vi "checkAllBridgesTested.vi"(8 "error in (no error)":errorcluster, 11 "TestMonitor in":refnum<class "TestMonitor.lvclass">) -> (0 "error out":errorcluster, 2 "allBridgesTestedIsTrue":bool, 3 "TestMonitor out":refnum<class "TestMonitor.lvclass">)   [LabVIEW 2013, in "TestMonitor.lvclass"]
uses:
  TestMonitor.lvclass
  TestMonitor.lvclass/TestMonitor.ctl
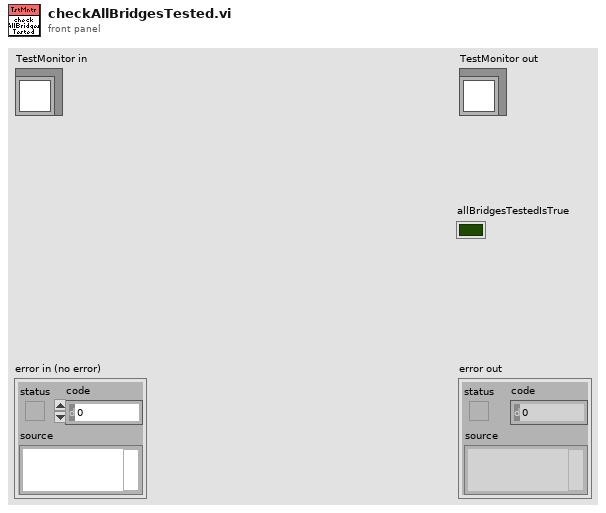
[diagram p1: front panel]
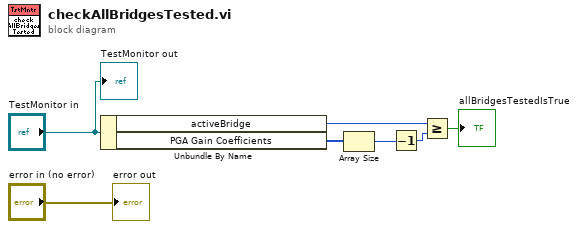
[diagram p0: block diagram]
diagram:
  n1 = Unbundle By Name("TestMonitor in") -> ("activeBridge"=w3:u32, "PGA Gain Coefficients"=w5:u8[])
  n2 = Array Size(array=w5) -> (size(s)=w4:i32)
  n3 = Decrement(x=w4) -> (x-1=w2:i32)
  n4 = Greater Or Equal?(x=w3, y=w2) -> (x >= y?=→"allBridgesTestedIsTrue":bool)
  "error out" <- "error in (no error)"
  "TestMonitor out" <- "TestMonitor in"
